vi "View VIs in Memory_82.vi"() -> ()   [LabVIEW 2011]
panel:
  out "Vis":i32
  in  "Get Modified":bool
  out "value":string[](array[string])
  in  "Get Callers":bool
  in  "Close FP":bool
  in  "Refresh List":bool
  in  "Abort":bool
  in  "Open":bool
  out "error out":errorcluster
  in  "Kill BUtton":bool
  in  "Done Button":bool
  in  "VI's in Memory":i32(listbox)
  in  "Paths of VIs in Memory":i32(listbox)
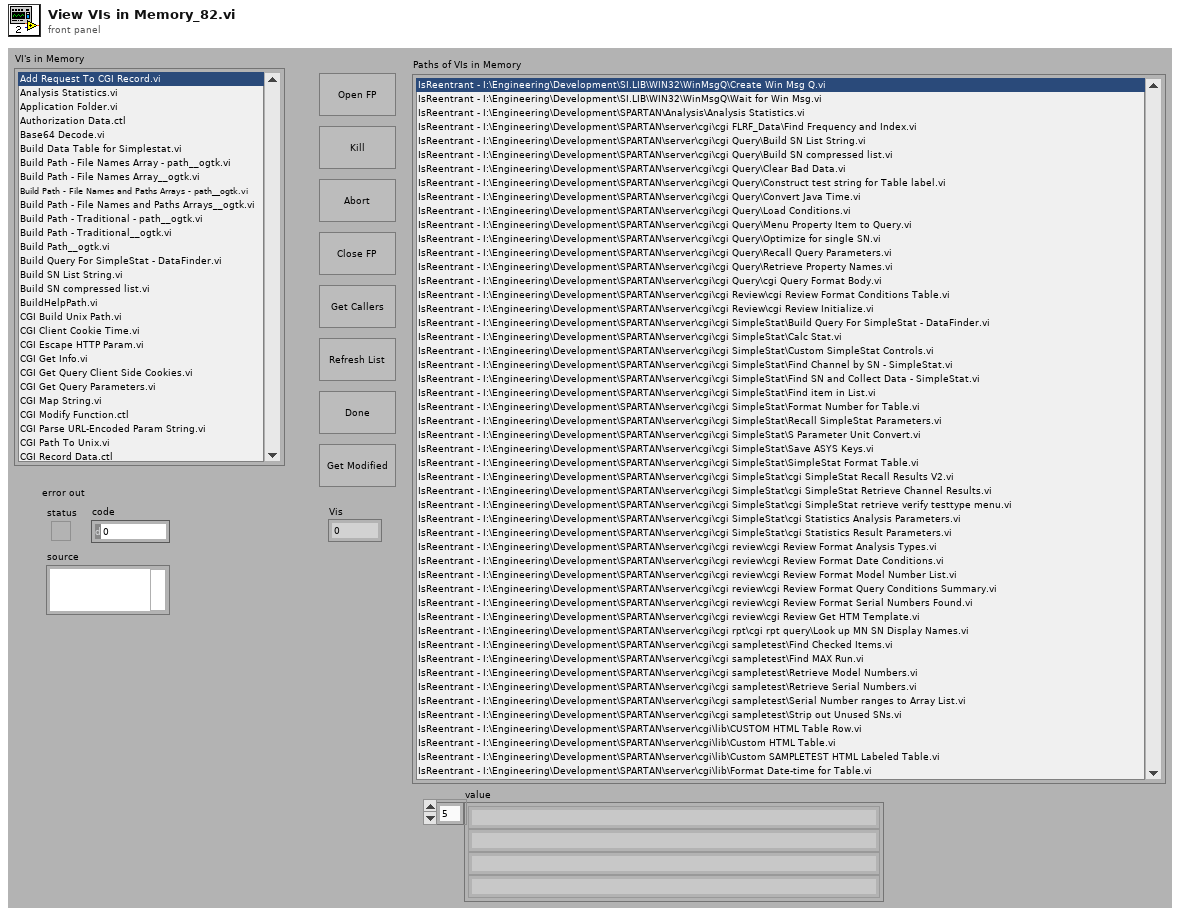
[diagram p1: front panel]
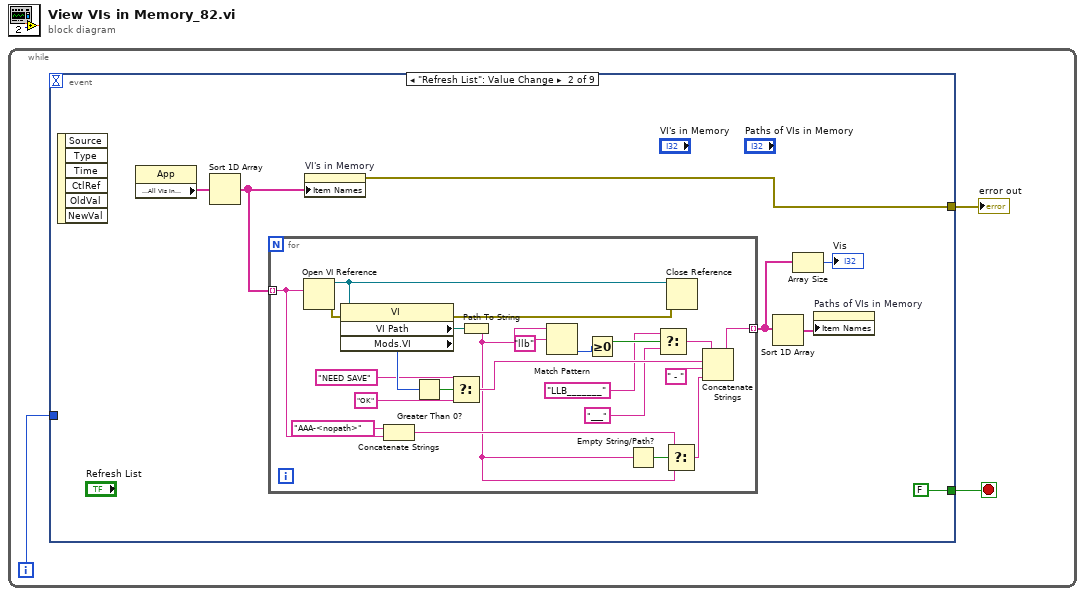
[diagram p0: block diagram]
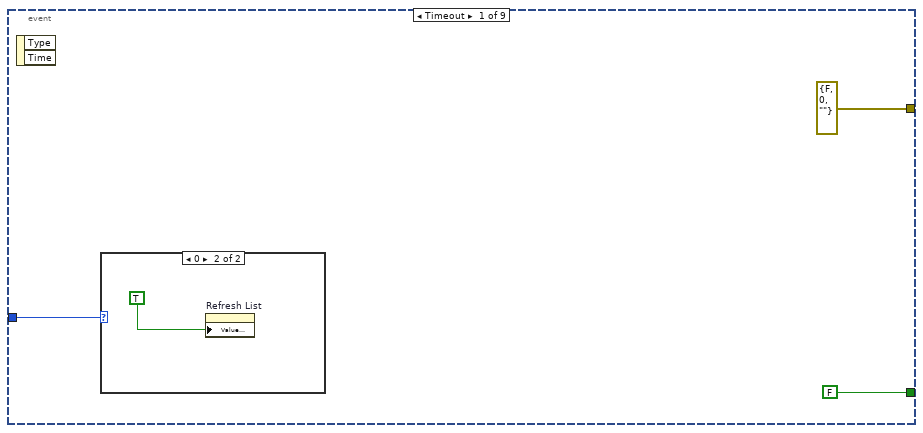
[diagram p2: hidden frame]
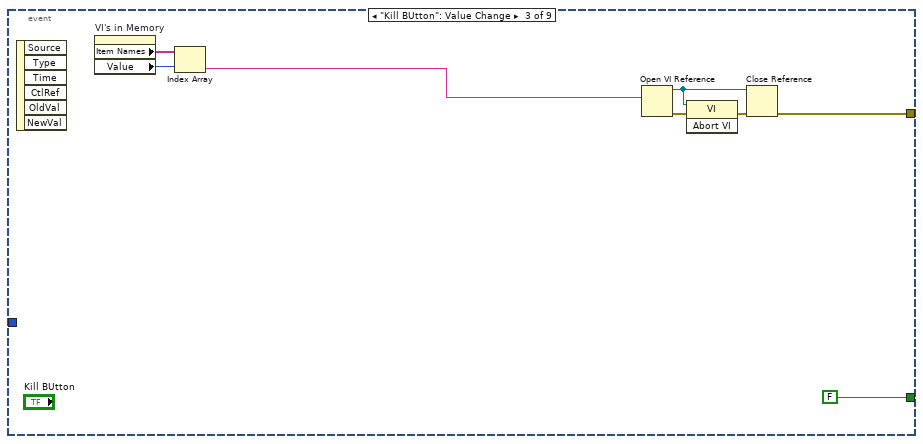
[diagram p4: hidden frame]
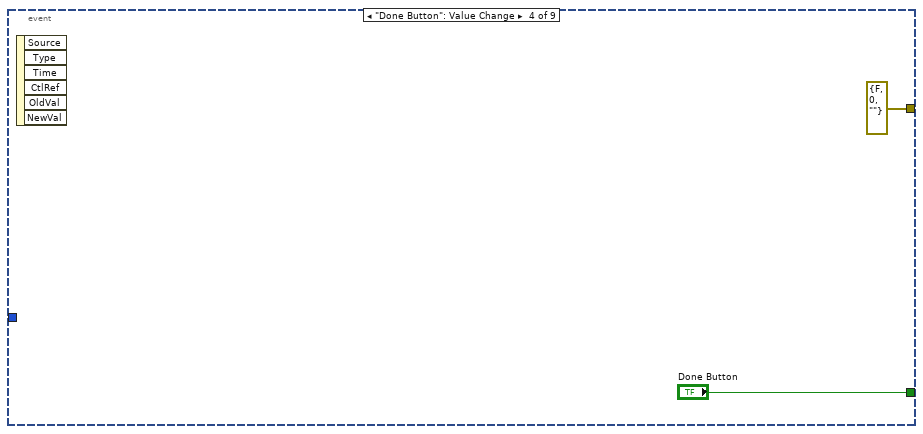
[diagram p5: hidden frame]
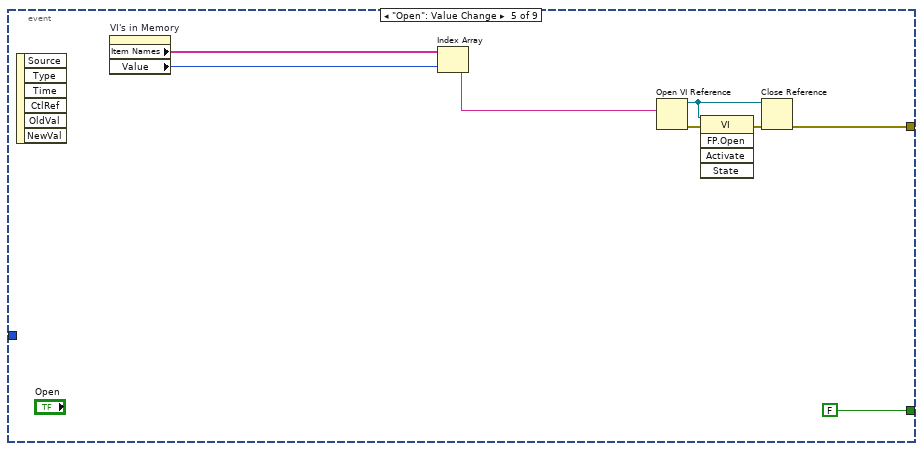
[diagram p6: hidden frame]
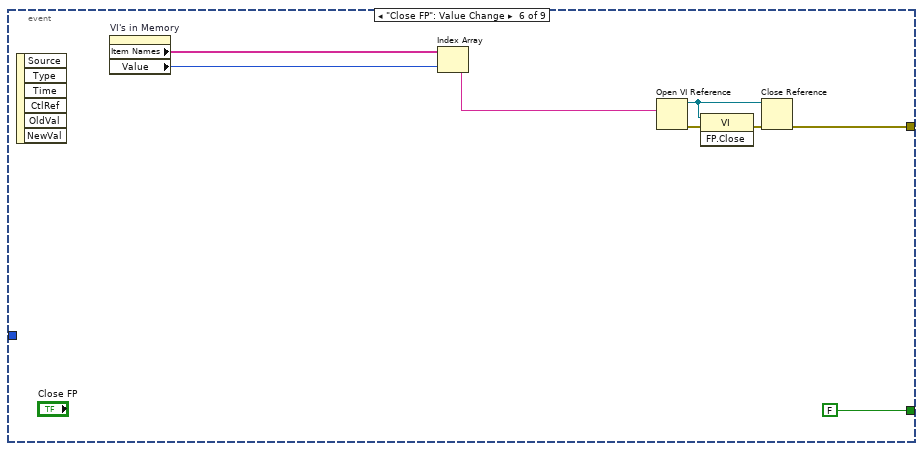
[diagram p7: hidden frame]
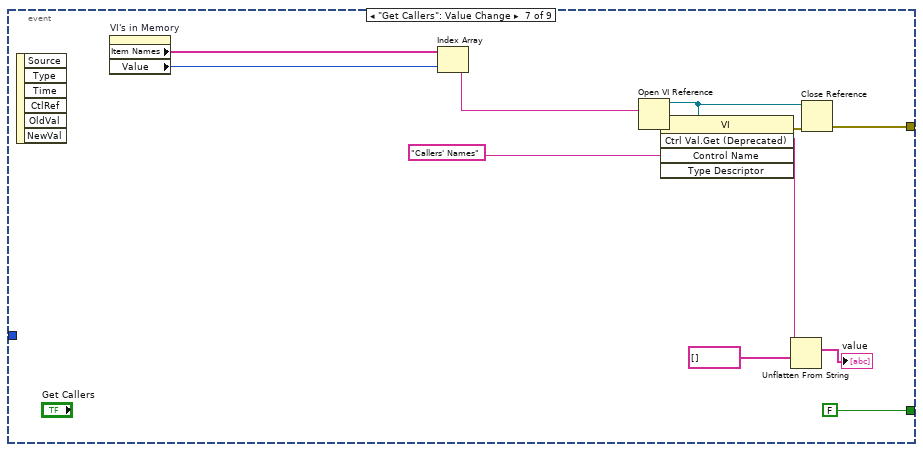
[diagram p8: hidden frame]
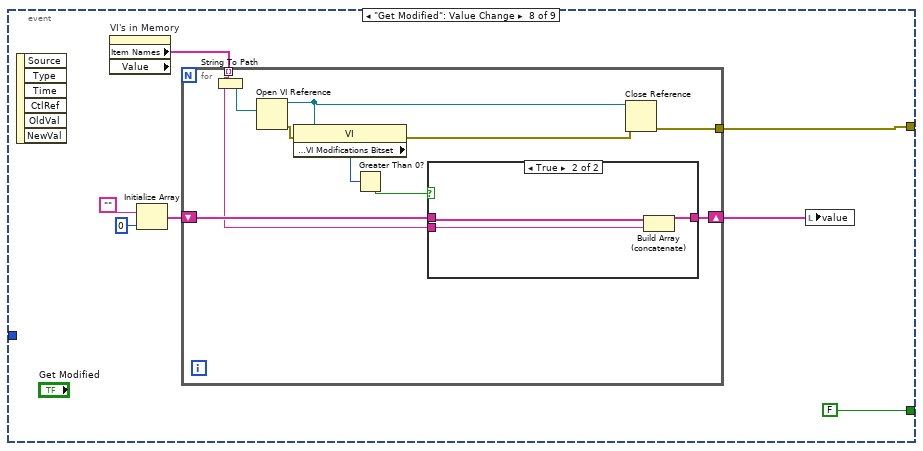
[diagram p9: hidden frame]
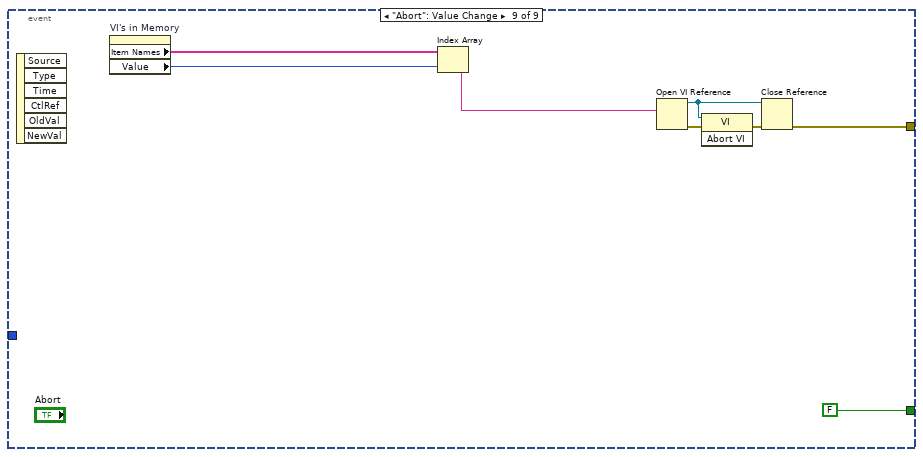
[diagram p11: hidden frame]
diagram:
  n1 = while {
    i -> [w2]
    stop <- w3 stop-if-true
    n2 = event shown="[1] \"Refresh List\": Value Change" {
      selector: _ -> [_ _ _ _ _ _ _ _ _]
      dyn-events: _ -> [_ _ _ _ _ _ _ _ _]
      timeout: _ -> [_ _ _ _ _ _ _ _ _]
      tunnel: [errorcluster {"status"=FALSE, "code"=0, "source"=""} ("error out") w10 w38 errorcluster {"status"=FALSE, "code"=0, "source"=""} ("error out") w48 w56 w64 w82 w97] -> w1
      tunnel: [FALSE ("Done Button") FALSE ("Done Button") FALSE ("Done Button") "Done Button" FALSE ("Done Button") FALSE ("Done Button") FALSE ("Done Button") FALSE ("Done Button") FALSE ("Done Button")] -> w3
      tunnel: w2 -> [w5 _ _ _ _ _ _ _ _]
      event Timeout {
        n3 = event-data() -> ()  [unwired: 3 out]
        n4 = case shown="0" w5 {
          frame Default {
          }
          frame 0 {
            n5 = property on="Refresh List" class="Bool"("Value (Signaling)"=TRUE) -> ()  [unwired: 2 in, 2 out]
          }
        }
      }
      event "Refresh List": Value Change {
        n6 = event-data() -> ()  [unwired: 7 out]
        n7 = property class="App"() -> ("Application:All VIs In Memory"=w14:string[])  [unwired: 2 in, 2 out]
        n8 = Sort 1D Array(array=w14) -> (sorted array=w12:string[])
        n9 = for {
          tunnel: w12 -> [w32] mode=indexing
          tunnel: [w23] -> w9 mode=indexing
          n10 = Open VI Reference(vi path=w32) -> (vi reference=w37:refnum<vi>, error out=w36:errorcluster)  [unwired: 1 in, 4 out]
          n11 = property class="VI"(reference=w37, error in=w36) -> (error out=w35:errorcluster, "VI Path"=w34:path, "Mods.VI"=w29:u32)  [unwired: 1 out]
          n12 = Concatenate Strings("AAA-<nopath>" ("string"), w32) -> (w30:string)
          n13 = Greater Than 0?(x=w29) -> (x > 0?=w15:bool)
          n14 = Select(t="NEED SAVE" ("string"), s=w15, f="OK" ("string")) -> (s? t:f=w26:string)
          n15 = Path To String(path=w34) -> (string=w22:string)
          n16 = Match Pattern(string=w22, regular expression="llb" ("string")) -> (offset past match=w19:i32)  [unwired: 4 out]
          n17 = Greater Or Equal To 0?(x=w19) -> (x >= 0?=w20:bool)
          n18 = Empty String/Path?(string/path=w22) -> (empty?=w33:bool)
          n19 = Select(t="LLB_______" ("string"), s=w20, f="___" ("string")) -> (s? t:f=w16:string)
          n20 = Select(t=w30, s=w33, f=w22) -> (s? t:f=w25:string)
          n21 = Close Reference(reference=w37, error in (no error)=w35) -> ()  [unwired: 1 out]
          n22 = Concatenate Strings(w16, w26, " - " ("string"), w25) -> (w23:string)
        }
        n23 = property on="VI's in Memory" class="LstBox (strict)"("Item Names"=w12) -> (error out=w10:errorcluster)  [unwired: 2 in, 1 out]
        n24 = Sort 1D Array(array=w9) -> (sorted array=w11:string[])
        n25 = Array Size(array=w9) -> (size(s)=→"Vis":i32)
        n26 = property on="Paths of VIs in Memory" class="LstBox (strict)"("Item Names"=w11) -> ()  [unwired: 2 in, 2 out]
      }
      event "Kill BUtton": Value Change {
        n27 = event-data() -> ()  [unwired: 7 out]
        n28 = property on="VI's in Memory" class="LstBox (strict)"() -> ("Item Names"=w45:string[], "Value"=w44:i32)  [unwired: 2 in, 2 out]
        n29 = Index Array(array=w45, index=w44) -> (element=w43:string)
        n30 = Open VI Reference(vi path=w43) -> (vi reference=w42:refnum<vi>, error out=w41:errorcluster)  [unwired: 1 in, 4 out]
        n31 = invoke class="VI" method="Abort VI"(reference=w42, error in=w41) -> (error out=w40:errorcluster)  [unwired: 1 in, 2 out]
        n32 = Close Reference(reference=w42, error in (no error)=w40) -> (error out=w38:errorcluster)
      }
      event "Done Button": Value Change {
        n33 = event-data() -> ()  [unwired: 7 out]
      }
      event "Open": Value Change {
        n34 = event-data() -> ()  [unwired: 7 out]
        n35 = property on="VI's in Memory" class="LstBox (strict)"() -> ("Item Names"=w55:string[], "Value"=w54:i32)  [unwired: 2 in, 2 out]
        n36 = Index Array(array=w55, index=w54) -> (element=w53:string)
        n37 = Open VI Reference(vi path=w53) -> (vi reference=w52:refnum<vi>, error out=w51:errorcluster)  [unwired: 1 in, 4 out]
        n38 = invoke class="VI" method="FP.Open"(reference=w52, error in=w51) -> (error out=w50:errorcluster)  [unwired: 3 in, 4 out]
        n39 = Close Reference(reference=w52, error in (no error)=w50) -> (error out=w48:errorcluster)
      }
      event "Close FP": Value Change {
        n40 = event-data() -> ()  [unwired: 7 out]
        n41 = property on="VI's in Memory" class="LstBox (strict)"() -> ("Item Names"=w63:string[], "Value"=w62:i32)  [unwired: 2 in, 2 out]
        n42 = Index Array(array=w63, index=w62) -> (element=w61:string)
        n43 = Open VI Reference(vi path=w61) -> (vi reference=w60:refnum<vi>, error out=w59:errorcluster)  [unwired: 1 in, 4 out]
        n44 = invoke class="VI" method="FP.Close"(reference=w60, error in=w59) -> (error out=w58:errorcluster)  [unwired: 1 in, 2 out]
        n45 = Close Reference(reference=w60, error in (no error)=w58) -> (error out=w56:errorcluster)
      }
      event "Get Callers": Value Change {
        n46 = event-data() -> ()  [unwired: 7 out]
        n47 = property on="VI's in Memory" class="LstBox (strict)"() -> ("Item Names"=w75:string[], "Value"=w74:i32)  [unwired: 2 in, 2 out]
        n48 = Index Array(array=w75, index=w74) -> (element=w73:string)
        n49 = Open VI Reference(vi path=w73) -> (vi reference=w66:refnum<vi>, error out=w72:errorcluster)  [unwired: 1 in, 4 out]
        n50 = invoke class="VI" method="Ctrl Val.Get (Deprecated)"(reference=w66, error in=w72, "Control Name"="Callers' Names") -> (error out=w71:errorcluster, "Get Control Value"=w68:string)  [unwired: 2 in, 3 out]
        n51 = Unflatten From String(type=string[] [] ("Callers' Names"), binary string=w68) -> (value=→"value":string[])  [unwired: 1 in, 4 out]
        n52 = Close Reference(reference=w66, error in (no error)=w71) -> (error out=w64:errorcluster)
      }
      event "Get Modified": Value Change {
        n53 = event-data() -> ()  [unwired: 7 out]
        n54 = property on="VI's in Memory" class="LstBox (strict)" props=["Item Names", "Value"]() -> ("Item Names"=w77:string[])  [unwired: 2 in, 3 out]
        n55 = Initialize Array("", 0 ("dimension size")) -> (w80:string[])
        n56 = for {
          tunnel: [w92] -> w82
          shift-right: [w84] -> w76
          shift-left: w80 -> [w85]
          tunnel: w77 -> [w83] mode=indexing
          n57 = String To Path(string=w83) -> (path=w87:path)
          n58 = Open VI Reference(vi path=w87) -> (vi reference=w91:refnum<vi>, error out=w90:errorcluster)  [unwired: 2 in, 3 out]
          n59 = property class="VI"(reference=w91, error in=w90) -> (error out=w89:errorcluster, "Modifications:VI Modifications Bitset"=w88:u32)  [unwired: 1 out]
          n60 = Greater Than 0?(x=w88) -> (x > 0?=w86:bool)
          n61 = case shown="True" w86 {
            tunnel: [w93 w94] -> w84
            tunnel: w85 -> [w93 w96]
            tunnel: w83 -> [_ w95]
            frame False {
            }
            frame True {
              n62 = Build Array (concatenate)(w96, w95) -> (w94:string[])
            }
          }
          n63 = Close Reference(reference=w91, error in (no error)=w89) -> (error out=w92:errorcluster)
        }
        n64 = local write "value"(w76) -> ()
      }
      event "Abort": Value Change {
        n65 = event-data() -> ()  [unwired: 7 out]
        n66 = property on="VI's in Memory" class="LstBox (strict)"() -> ("Item Names"=w104:string[], "Value"=w103:i32)  [unwired: 2 in, 2 out]
        n67 = Index Array(array=w104, index=w103) -> (element=w102:string)
        n68 = Open VI Reference(vi path=w102) -> (vi reference=w101:refnum<vi>, error out=w100:errorcluster)  [unwired: 1 in, 4 out]
        n69 = invoke class="VI" method="Abort VI"(reference=w101, error in=w100) -> (error out=w99:errorcluster)  [unwired: 1 in, 2 out]
        n70 = Close Reference(reference=w101, error in (no error)=w99) -> (error out=w97:errorcluster)
      }
    }
    "error out" <- w1
  }
